vi "test Parse Sorted Object Dictionary_3.vi"(11 "Test Case In":refnum<class "test Electronic Datasheet.lvclass">) -> (0 "error out":errorcluster, 3 "Test Case Out":refnum<class "test Electronic Datasheet.lvclass">)   [LabVIEW 2024, in "test Electronic Datasheet.lvclass"]
uses:
  test Electronic Datasheet.lvclass
  C:/Program Files/National Instruments/LabVIEW 2024/vi.lib/Astemes/LUnit/Test Case.lvclass
  Core/Object Type.ctl
  <vilib>/Astemes/LUnit/Test Case.lvclass/Test Case.ctl
  <vilib>/Astemes/LUnit/Append Fail Result.vi
  <vilib>/Astemes/LUnit/Append Pass Result.vi
  <vilib>/Astemes/LUnit/Run In UI.vi
  <vilib>/Utility/error.llb/Clear Errors.vi
  Electronic Datasheet/utils/Electronic Datasheet_GetAttributes.vi
  Electronic Datasheet/Electronic Datasheet.lvclass
  <vilib>/Astemes/LUnit/Test Case.lvclass
  Core/Electronic Datasheet.lvlib
  Core/OD Entry/OD Entry.lvclass
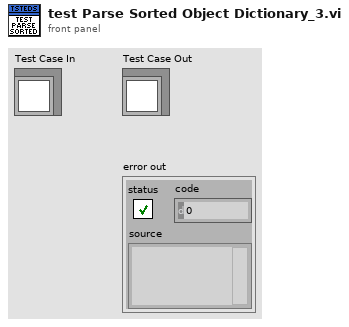
[diagram p1: front panel]
types:
  T1 = typedef "Electronic Datasheet.lvlib/Object Type.ctl" = u8
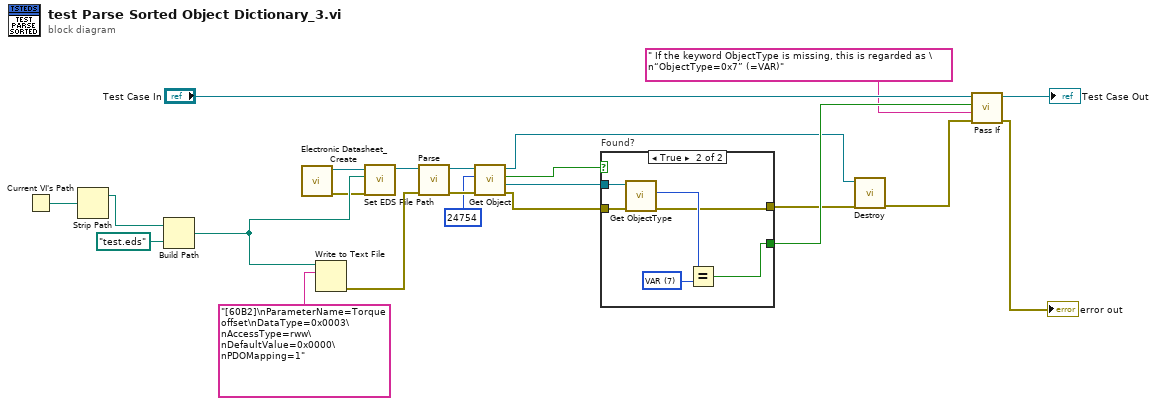
[diagram p0: block diagram]
diagram:
  n1 = Current VI's Path() -> (path=w19:path)
  n2 = Strip Path(path=w19) -> (stripped path=w15:path)  [unwired: 1 out]
  n3 = Build Path(base path=w15, name or relative path=path "test.eds") -> (appended path=w16:path)
  n4 = call "Electronic Datasheet_Create.vi"() -> ("Error Out"=w8:errorcluster, "reference out"=w7:refnum<class "Electronic Datasheet.lvclass">)  [unwired: 10 in]
  n5 = Write to Text File(file (use dialog)=w16, text="[60B2]\nParameterName=Torque offset\nDataType=0x0003\nAccessType=rww\nDefaultValue=0x0000\nPDOMapping=1") -> (error out=w17:errorcluster)  [unwired: 2 in, 2 out]
  n6 = call "Set EDS File Path.vi"("error in"=w8, "EDS File Path"=w16, "reference in"=w7) -> ("reference out"=w20:refnum<class "Electronic Datasheet.lvclass">)  [unwired: 7 in, 1 out]
  n7 = call "Parse.vi"("error in"=w17, "reference in"=w20) -> ("error out"=w6:errorcluster, "reference out"=w14:refnum<class "Electronic Datasheet.lvclass">)  [unwired: 8 in]
  n8 = call "Get Object.vi"("error in"=w6, "Index"=u16 24754, "reference in"=w14) -> ("error out"=w5:errorcluster, "OD Entry"=w3:refnum<class "OD Entry.lvclass">, "Found?"=w4:bool, "reference out"=w2:refnum<class "Electronic Datasheet.lvclass">)  [unwired: 5 in]
  n9 = case "Found?" shown="True" w4 {
    selector: w4 -> [w24 _]
    tunnel: w3 -> [_ w31]
    tunnel: w5 -> [w25 w30]
    tunnel: [w24 w26] -> w12
    tunnel: [w25 w27] -> w10
    frame False {
    }
    frame True {
      w28 = T1 7 items=["NULL"=0, "DOMAIN"=2, "DEFTYPE"=5, "DEFSTRUCT"=6, "VAR"=7, "ARRAY"=8, "RECORD"=9] ("y")
      n10 = call "Get ObjectType.vi"("Error In"=w30, "reference in"=w31) -> ("Error Out"=w27:errorcluster, "ObjectType"=w29:T1)  [unwired: 7 in, 1 out]
      n11 = Equal?(x=w29, y=w28) -> (x = y?=w26:bool)
    }
  }
  n12 = call-dynamic "Destroy.vi"("Error In"=w10, "reference in"=w2) -> ("Error Out"=w11:errorcluster)  [unwired: 8 in, 1 out]
  n13 = call <vilib>:"Pass If.vi"("error in (no error)"=w11, "Message"=" If the keyword ObjectType is missing, this is regarded as \n“ObjectType=0x7” (=VAR)", "Pass?"=w12, "LUnit Test Case In"="Test Case In") -> ("error out"=→"error out":errorcluster, "LUnit Test Case Out"=→"Test Case Out":refnum<class "test Electronic Datasheet.lvclass">)  [unwired: 6 in]
